vi "ProdaNG.Tree.WabcoPart.Open.vi"(7 "Tree":refnum<vi>, 8 "error in (no error)":errorcluster, 10 "Tag":string) -> (0 "error out":errorcluster)   [LabVIEW 2016]
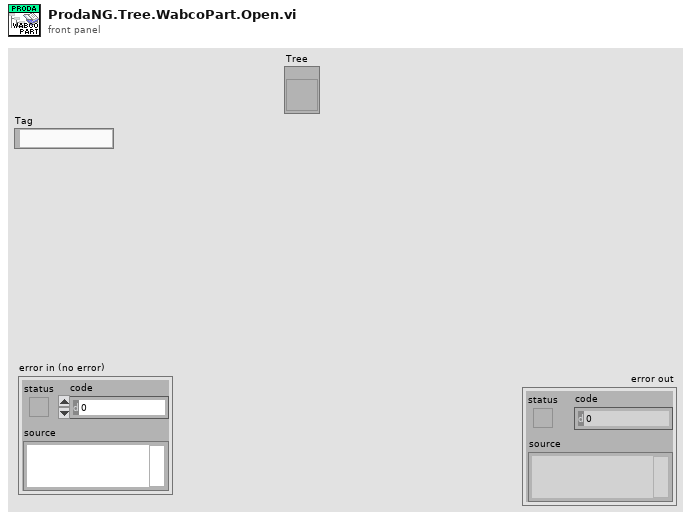
[diagram p1: front panel]
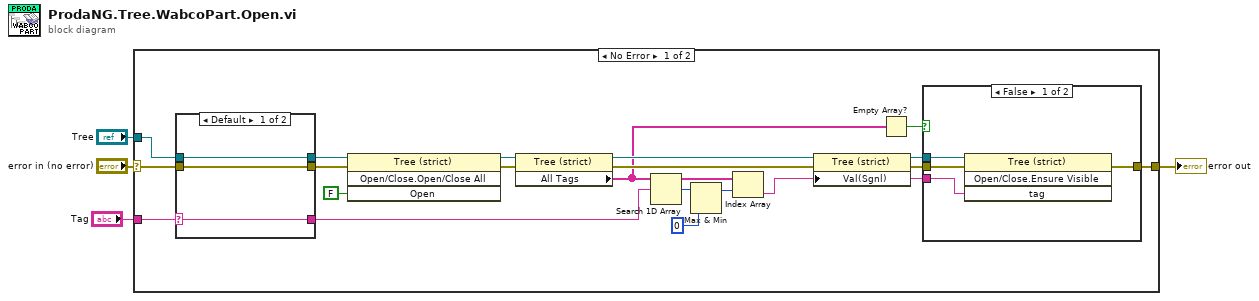
[diagram p0: block diagram]
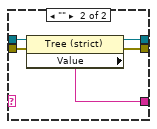
[diagram p3: hidden frame]
diagram:
  n1 = case shown="No Error" "error in (no error)" {
    selector: "error in (no error)" -> [w14 w38]
    tunnel: [w10 w38] -> w3
    tunnel: "Tree" -> [w11 _]
    tunnel: "Tag" -> [w9 _]
    frame No Error {
      n2 = case shown="Default" w9 {
        selector: w9 -> [w32 _]
        tunnel: w14 -> [w30 w37]
        tunnel: [w30 w36] -> w13
        tunnel: [w31 w35] -> w12
        tunnel: w11 -> [w31 w34]
        tunnel: [w32 w33] -> w8
        frame Default {
        }
        frame "" {
          n3 = property class="Tree (strict)"(reference=w34, error in=w37) -> (reference out=w35:refnum<vi>, error out=w36:errorcluster, "Value"=w33:string)
        }
      }
      n4 = invoke class="Tree (strict)" method="Open/Close.Open/Close All"(reference=w12, error in=w13, "Open"=FALSE ("Open?")) -> (reference out=w18:refnum<vi>, error out=w17:errorcluster)  [unwired: 1 in, 2 out]
      n5 = property class="Tree (strict)"(reference=w18, error in=w17) -> (reference out=w16:refnum<vi>, error out=w15:errorcluster, "All Tags"=w5:string[])
      n6 = Search 1D Array(1D array=w5, element=w8) -> (index of element=w22:i32)  [unwired: 1 in]
      n7 = Max & Min(x=w22, y=0) -> (max(x,y)=w20:i32)  [unwired: 1 out]
      n8 = Index Array(array=w5, index=w20) -> (element=w7:string)
      n9 = property class="Tree (strict)"(reference=w16, error in=w15, "Val(Sgnl)"=w7) -> (reference out=w23:refnum<vi>, error out=w24:errorcluster)
      n10 = Empty Array?(array=w5) -> (empty?=w6:bool)
      n11 = case shown="False" w6 {
        tunnel: w24 -> [w28 w29]
        tunnel: w23 -> [w27 _]
        tunnel: [w26 w29] -> w10
        tunnel: w7 -> [w25 _]
        frame False {
          n12 = invoke class="Tree (strict)" method="Open/Close.Ensure Visible"(reference=w27, error in=w28, "tag"=w25) -> (error out=w26:errorcluster)  [unwired: 1 in, 3 out]
        }
        frame True {
        }
      }
    }
    frame Error {
    }
  }
  "error out" <- w3
